vi "Simple_Bool.vi"() -> ()   [LabVIEW 2021]
panel:
  out "lamp":bool
  in  "start_PB":bool
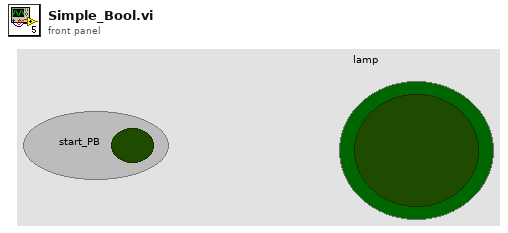
[diagram p1: front panel]
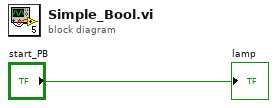
[diagram p0: block diagram]
diagram:
  "lamp" <- "start_PB"
